vi "Analyze.vi"(8 "Error In":errorcluster, 10 "Treshold (rms)":dbl, 11 "N-Channel Data (2D DBL)":dbl[][](array[numeric])) -> (0 "Error Out":errorcluster, 1 "Message":string, 2 "Threshold exceeded?":bool, 3 "N-Channel Data RMS Results":dbl[](array[numeric]))   [LabVIEW 2020]
uses:
  <vilib>/Analysis/5stat.llb/RMS (DBL).vi
  <vilib>/Analysis/NI_AALPro.lvlib
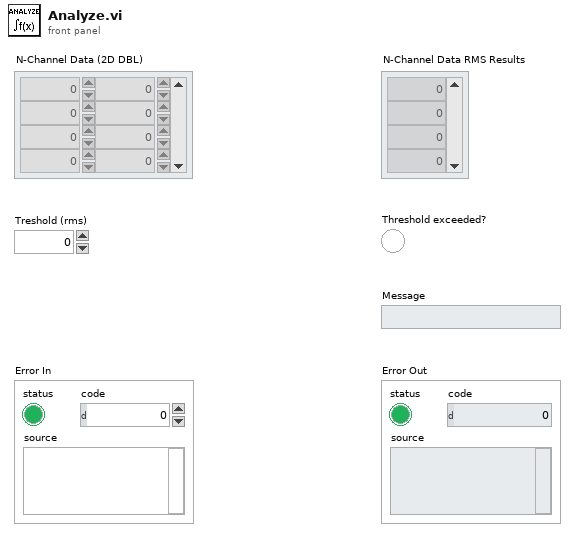
[diagram p1: front panel]
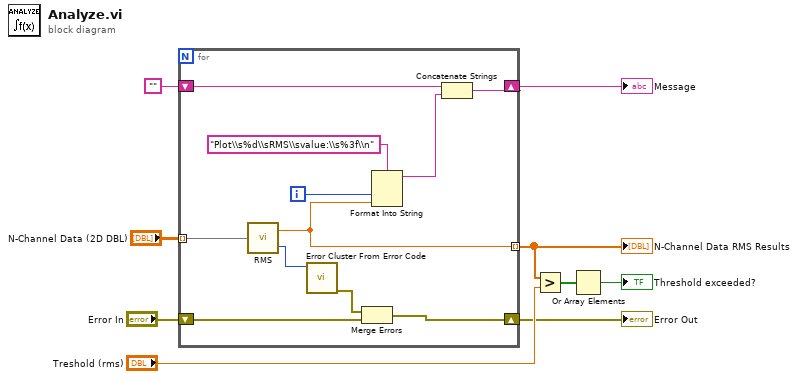
[diagram p0: block diagram]
diagram:
  n1 = for {
    tunnel: "N-Channel Data (2D DBL)" -> [w15] mode=indexing
    shift-right: [w16] -> w6
    shift-left: "" -> [w18]
    tunnel: [w14] -> w5 mode=indexing
    shift-right: [w10] -> w3
    shift-left: "Error In" -> [w11]
    i -> [w20]
    n2 = call-poly <vilib>:"RMS.vi"("X"=w15) -> ("rms value"=w14:dbl, "error"=w13:i32)
    n3 = call <vilib>:"Error Cluster From Error Code.vi"("error code (0)"=w13) -> ("error out"=w12:errorcluster)  [unwired: 8 in]
    n4 = Merge Errors(w12, w11) -> (w10:errorcluster)
    n5 = Format Into String(format string="Plot\\s%d\\sRMS\\svalue:\\s%3f\\n", w20, w14) -> (resulting string=w17:string)  [unwired: 2 in, 1 out]
    n6 = Concatenate Strings(w18, w17) -> (w16:string)
  }
  "Error Out" <- w3
  "N-Channel Data RMS Results" <- w5
  "Message" <- w6
  n7 = Greater?(x=w5, y="Treshold (rms)") -> (0:w2:bool[])
  n8 = Or Array Elements(Boolean array=w2) -> (logical OR=→"Threshold exceeded?":bool)
